vi "Get Configuration.vi"(8 "error in (no error)":errorcluster, 11 "DSF UDP Thread Configuration in":refnum<class "UDP Thread Configuration.lvclass">) -> (0 "error out":errorcluster, 2 "thread settings":T1, 3 "DSF UDP Thread Configuration out":refnum<class "UDP Thread Configuration.lvclass">)   [LabVIEW 2017, in "UDP.lvlib" / "UDP Thread Configuration.lvclass"]
uses:
  UDP Thread Configuration.lvclass
  Thread Settings.ctl
  UDP Thread Configuration.lvclass/UDP Thread Configuration.ctl
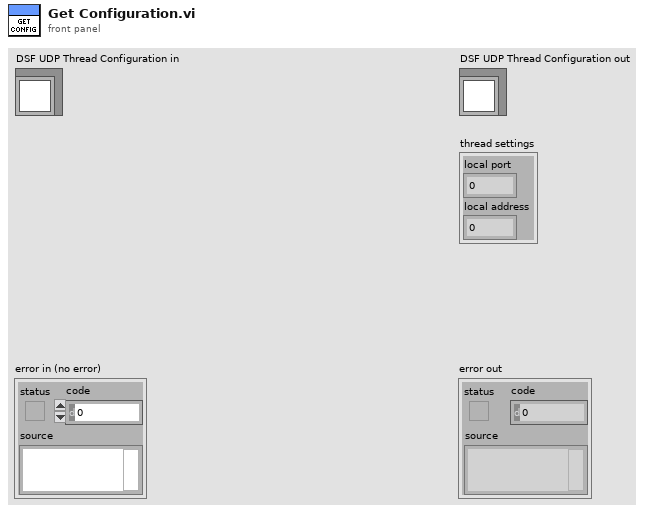
[diagram p1: front panel]
types:
  T1 = typedef "UDP.lvlib/UDP Thread Configuration.lvclass/Thread Settings.ctl" = cluster{"local port":u16, "local address":u32}
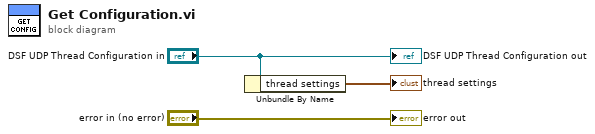
[diagram p0: block diagram]
diagram:
  n1 = Unbundle By Name("DSF UDP Thread Configuration in") -> ("thread settings"=→"thread settings":T1)
  "error out" <- "error in (no error)"
  "DSF UDP Thread Configuration out" <- "DSF UDP Thread Configuration in"
